vi "Lift to Angle Implementation.vi"(8 "Deadband (Power)":dbl, 10 "Angle Setpoint In":dbl, 11 "Hood":T1) -> (0 "Finished?":bool, 3 "Angle Setpoint Out":dbl)   [LabVIEW 2019]
uses:
  <vilib>/Rock Robotics/WPI/MotorControl/WPI_MotorControlDeviceRef.ctl
  <vilib>/Rock Robotics/WPI/MotorControl/WPI_MotorControlType.ctl
  <vilib>/Rock Robotics/SystemInterfaces/DIO/FPGA_DIOPWMChannel.ctl
  <vilib>/Rock Robotics/WPI/PWM/WPI_PWMDeadband.ctl
  <vilib>/Rock Robotics/SystemInterfaces/DIO/FPGA_DIOChannel.ctl
  Turret Published Globals.vi
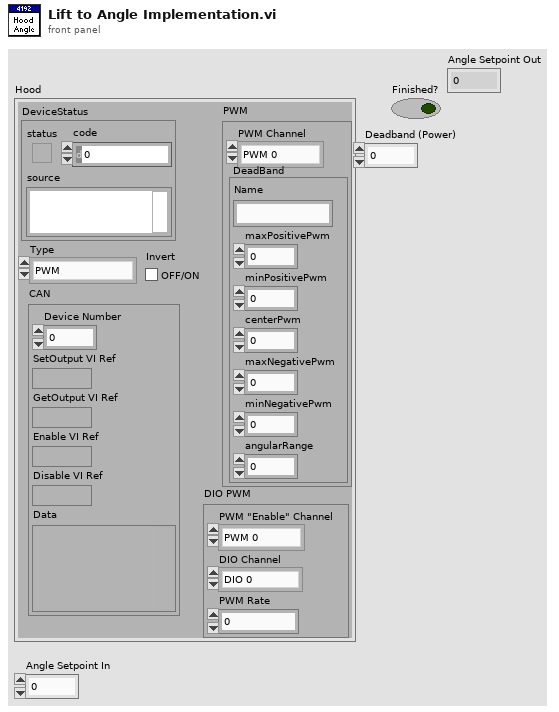
[diagram p1: front panel]
types:
  T1 = typedef "WPI_MotorControlDeviceRef.ctl" = cluster{"DeviceStatus":errorcluster, "Type":T2, "PWM":cluster{"PWM Channel":T3, "DeadBand":T4}, "CAN":cluster{"Device Number":u8, "SetOutput VI Ref":variant, "GetOutput VI Ref":variant, "Enable VI Ref":variant, "Disable VI Ref":variant, "Data":variant}, "Invert":bool, "DIO PWM":cluster{"PWM \"Enable\" Channel":T3, "DIOChannel":T5, "PWM Rate":dbl}}
  T2 = typedef "WPI_MotorControlType.ctl" = enum16{"PWM", "CAN", "DIO PWM"}
  T3 = typedef "FPGA_DIOPWMChannel.ctl" = enum8{"PWM 0", "PWM 1", "PWM 2", "PWM 3", "PWM 4", "PWM 5", "PWM 6", "PWM 7", "PWM 8", "PWM 9", "PWM MXP 0", "PWM MXP 1", "PWM MXP 2", "PWM MXP 3", "PWM MXP 4", "PWM MXP 5", "PWM MXP 6", "PWM MXP 7", "PWM MXP 8", "PWM MXP 9", "Invalid"}
  T4 = typedef "WPI_PWMDeadband.ctl" = cluster{"Name":string, "maxPositivePwm":i32, "minPositivePwm":i32, "centerPwm":i32, "maxNegativePwm":i32, "minNegativePwm":i32, "angularRange":u16}
  T5 = typedef "FPGA_DIOChannel.ctl" = enum8{"DIO 0", "DIO 1", "DIO 2", "DIO 3", "DIO 4", "DIO 5", "DIO 6", "DIO 7", "DIO 8", "DIO 9", "DIO MXP 0", "DIO MXP 1", "DIO MXP 2", "DIO MXP 3", "DIO MXP 4", "DIO MXP 5", "DIO MXP 6", "DIO MXP 7", "DIO MXP 8", "DIO MXP 9", "DIO MXP 10", "DIO MXP 11", "DIO MXP 12", "DIO MXP 13", "DIO MXP 14", "DIO MXP 15", "SPI Port CS1", "SPI Port CS2", "SPI Port CS3", "SPI Port MISO", "SPI Port MOSI", "Invalid"}
  T6 = cluster{"Shooter Velocity":cluster{"Sensor Velocity":dbl, "Setpoint":dbl, "Applied Output":dbl}, "Turret Position":cluster{"output":dbl, "Horizontal Offset":dbl}, "Hood Position":cluster{"Sensor Velocity":dbl, "Setpoint":dbl, "Applied Output":dbl}, "Shooter PID Constants":cluster{"P Gain":dbl, "I Gain":dbl, "D Gain":dbl, "F Gain":dbl, "I Zone":dbl, "Min Output":dbl, "Max Output":dbl}, "Hood PID Constants":cluster{"P Gain":dbl, "I Gain":dbl, "D Gain":dbl, "F Gain":dbl, "I Zone":dbl, "Min Output":dbl, "Max Output":dbl}, "Turret PID Constants":cluster{"P Gain":dbl, "I Gain":dbl, "D Gain":dbl, "F Gain":dbl, "I Zone":dbl, "Min Output":dbl, "Max Output":dbl}, "Limelight PID Gains":cluster{"proportional gain (Kc)":dbl, "integral time (Ti, min)":dbl, "derivative time (Td, min)":dbl}}
  T7 = cluster{"P Gain":dbl, "I Gain":dbl, "D Gain":dbl, "F Gain":dbl, "I Zone":dbl, "Min Output":dbl, "Max Output":dbl}
  T8 = cluster{"Sensor Position":dbl, "Angle Setpoint In":dbl, "Applied Output":dbl}
  T9 = cluster{"Shooter Up To Speed?":bool, "Aligned With Target?":bool, "Hood at Angle?":bool, "Shooting?":bool, "Hood Angle":dbl, "Turret Angle":dbl}
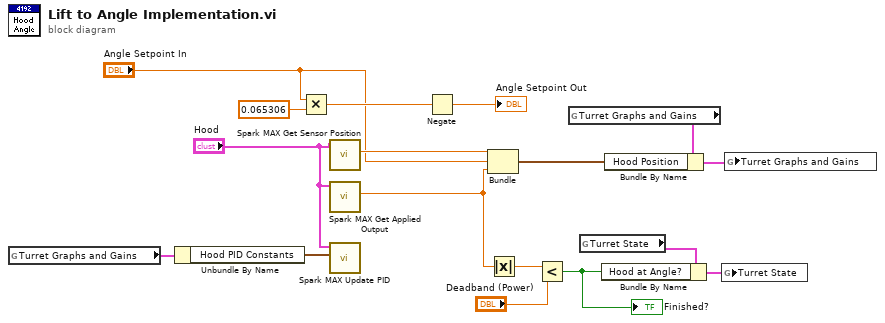
[diagram p0: block diagram]
diagram:
  n1 = global read "Turret Published Globals.vi" "Turret Graphs and Gains"() -> (w13:T6)
  n2 = Unbundle By Name(w13) -> ("Hood PID Constants"=w12:T7)
  n3 = Multiply(x="Angle Setpoint In", y=0.065306) -> (x*y=w14:dbl)
  n4 = call <vilib>:"Spark MAX Get Sensor Position.vi"("MotorControlDevRef in"="Hood") -> ("Sensor Position"=w16:dbl)  [unwired: 7 in, 3 out]
  n5 = call <vilib>:"Spark MAX Get Applied Output.vi"("MotorControlDevRef in"="Hood") -> ("Applied Output"=w10:dbl)  [unwired: 7 in, 3 out]
  n6 = call "Spark MAX Update PID.vi"("MotorControlDeviceRef"="Hood", "PID Constants"=w12) -> ()  [unwired: 8 in]
  n7 = Negate(x=w14) -> (-x=→"Angle Setpoint Out":dbl)
  n8 = Bundle("Sensor Position"=w16, "Angle Setpoint In"="Angle Setpoint In", "Applied Output"=w10) -> (w2:T8)  [unwired: 1 in]
  n9 = Absolute Value(x=w10) -> (abs(x)=w15:dbl)
  n10 = Less?(x=w15, y="Deadband (Power)") -> (x < y?=w6:bool)
  "Finished?" <- w6
  n11 = global read "Turret Published Globals.vi" "Turret Graphs and Gains"() -> (w3:T6)
  n12 = global read "Turret Published Globals.vi" "Turret State"() -> (w8:T9)
  n13 = Bundle By Name(cluster=w8, "Hood at Angle?"=w6) -> (w5:T9)
  n14 = Bundle By Name(cluster=w3, "Hood Position"=w2) -> (w4:T6)
  n15 = global write "Turret Published Globals.vi" "Turret State"(w5) -> ()
  n16 = global write "Turret Published Globals.vi" "Turret Graphs and Gains"(w4) -> ()
